vi "Append Pose.vi"(8 "error in (no error)":errorcluster, 10 "serial arm pose":T1, 11 "serial arm in":refnum<class "NI_Robotics_Serial Robot Arm.lvclass">) -> (0 "error out":errorcluster, 3 "serial arm out":refnum<class "NI_Robotics_Serial Robot Arm.lvclass">)   [LabVIEW 2017, in "NI_Robotics_Serial Robot Arm.lvclass"]
uses:
  <vilib>/robotics/Kinematics/Robot/NI_Robotics_Serial Robot Arm.lvclass
  <vilib>/robotics/Kinematics/Robot/Robot Pose.ctl
  <vilib>/robotics/Kinematics/Robot/NI_Robotics_Serial Robot Arm.lvclass/NI_Robotics_Serial Robot Arm.ctl
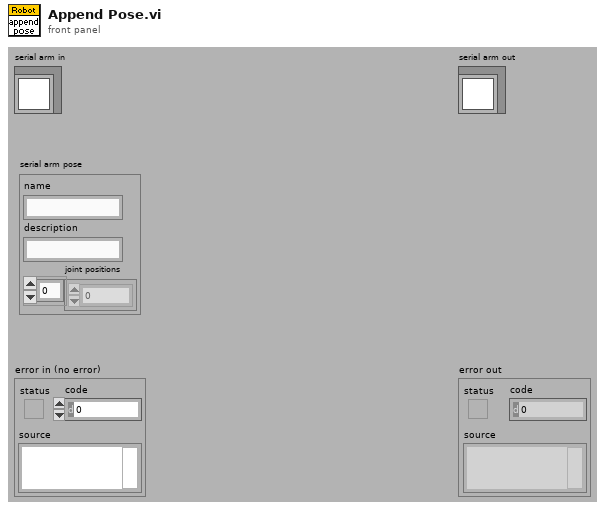
[diagram p1: front panel]
types:
  T1 = typedef "NI_Robotics_Serial Robot Arm.lvclass/Robot Pose.ctl" = cluster{"name":string, "description":string, "joint positions":dbl[]}
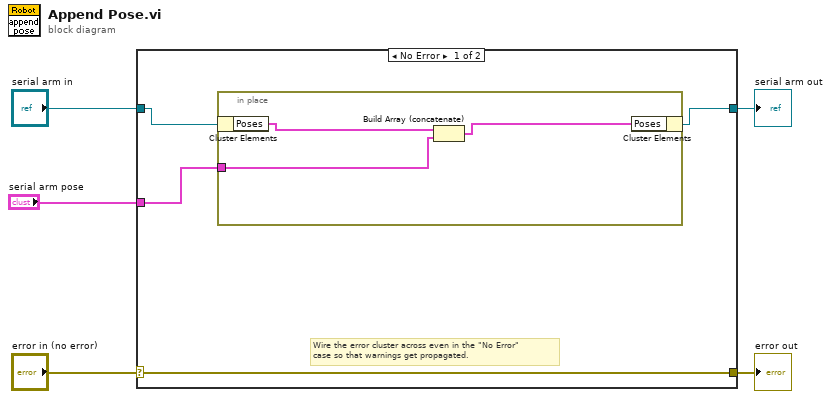
[diagram p0: block diagram]
diagram:
  n1 = case shown="No Error" "error in (no error)" {
    selector: "error in (no error)" -> [w9 w14]
    tunnel: [w9 w14] -> w4
    tunnel: [w7 w13] -> w2
    tunnel: "serial arm in" -> [w8 w13]
    tunnel: "serial arm pose" -> [w6 _]
    frame No Error {
      # "Wire the error cluster across even in the \"No Error\"\ncase so that warnings get propagated."
      n2 = in-place {
        in-place-border: w6 -> [w12]
        n3 = in-place-cluster #1(w8) -> ("Poses"=w11:T1[])
        n4 = Build Array (concatenate)(w11, w12) -> (w10:T1[])
        n5 = in-place-cluster #1("Poses"=w10) -> (w7:refnum<class "NI_Robotics_Serial Robot Arm.lvclass">)
      }
    }
    frame Error {
    }
  }
  "error out" <- w4
  "serial arm out" <- w2
